vi "Receive Value Change Event.vi"(8 "error in (no error)":errorcluster, 10 "ValueChangeMsg":refnum<class "ValueChangeMsg.lvclass">, 11 "IViewable In":refnum<class "IViewable.lvclass">) -> (0 "error out":errorcluster, 3 "IViewable Out":refnum<class "IViewable.lvclass">)   [LabVIEW 2018, in "MVA Framework.lvlib" / "IViewable.lvlib" / "IViewable.lvclass"]
doc: "接收值更改事件"
uses:
  IViewable.lvclass
  <vilib>/ActorFramework/Actor/Actor.lvclass
  IViewable Messages/Catch Nested Value Change Msg/Nested Value Update Msg.lvclass
  ActorEvents/IEventAggregator Messages/ValueChangeMsg/ValueChangeMsg.lvclass
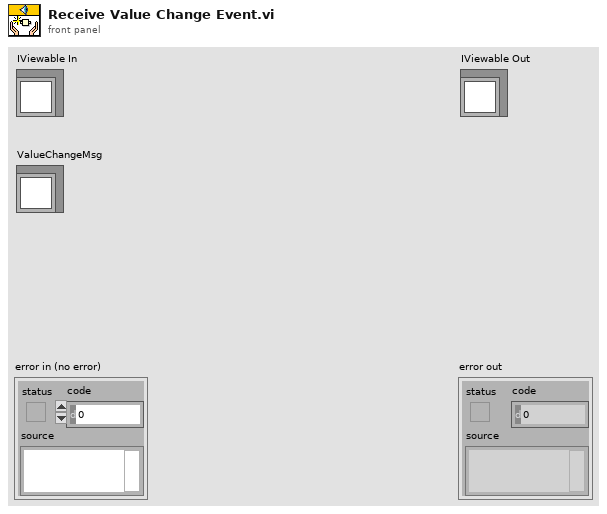
[diagram p1: front panel]
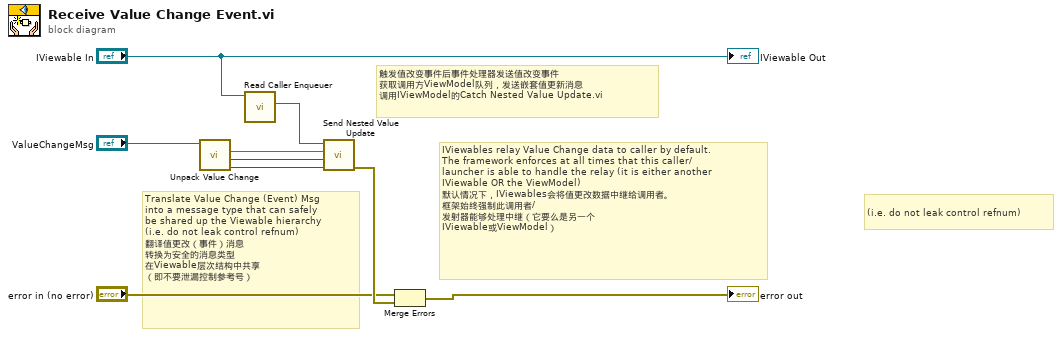
[diagram p0: block diagram]
diagram:
  # "触发值改变事件后事件处理器发送值改变事件\n获取调用方ViewModel队列，发送嵌套值更新消息\n调用IViewModel的Catch Nested Value Update.vi"
  # "(i.e. do not leak control refnum)"
  # "Translate Value Change (Event) Msg\ninto a message type that can safely\nbe shared up the Viewable hierarchy\n(i.e. do not leak control refnum)\n翻译值更改（事件）消息\n转换为安全的消息类型\n在Viewable层次结构中共享\n（即不要泄漏控制参考号）"
  # "IViewables relay Value Change data to caller by default.\nThe framework enforces at all times that this caller/\nlauncher is able to handle the relay (it is either another\nIViewable OR the ViewModel)\n默认情况下，IViewables会将值更改数据中继给调用者。\n框架始终强制此调用者/\n发射器能够处理中继（它要么是另一个\nIViewable或ViewModel）"
  n1 = call "Unpack Value Change.vi"("ValueChangeMsg"="ValueChangeMsg") -> ("New Value"=w1:variant, "Time"=w2:u32, "Control Label"=w3:string)  [unwired: 6 in, 2 out]
  n2 = call <vilib>:"Read Caller Enqueuer.vi"("Actor"="IViewable In") -> ("Caller Enqueuer"=w8:refnum<class "Message Enqueuer.lvclass">)  [unwired: 10 in]
  n3 = call "Send Nested Value Update.vi"("Value"=w1, "Time (Get Time)"=w2, "Datum Name"=w3, "Message Enqueuer"=w8) -> ("error out"=w9:errorcluster)  [unwired: 6 in, 1 out]
  n4 = Merge Errors("error in (no error)", w9) -> (→"error out":errorcluster)
  "IViewable Out" <- "IViewable In"
